vi "Diff_Drive_System_Dash_Write.vi"   [LabVIEW 2019]
uses:
  Diff_Drive_System_Globals.vi
  <vilib>/Rock Robotics/Network Tables/NT Write Numeric Array.vi
  <vilib>/Rock Robotics/Network Tables/NT Write Number.vi
  <vilib>/Rock Robotics/Network Tables/NT Write Boolean.vi
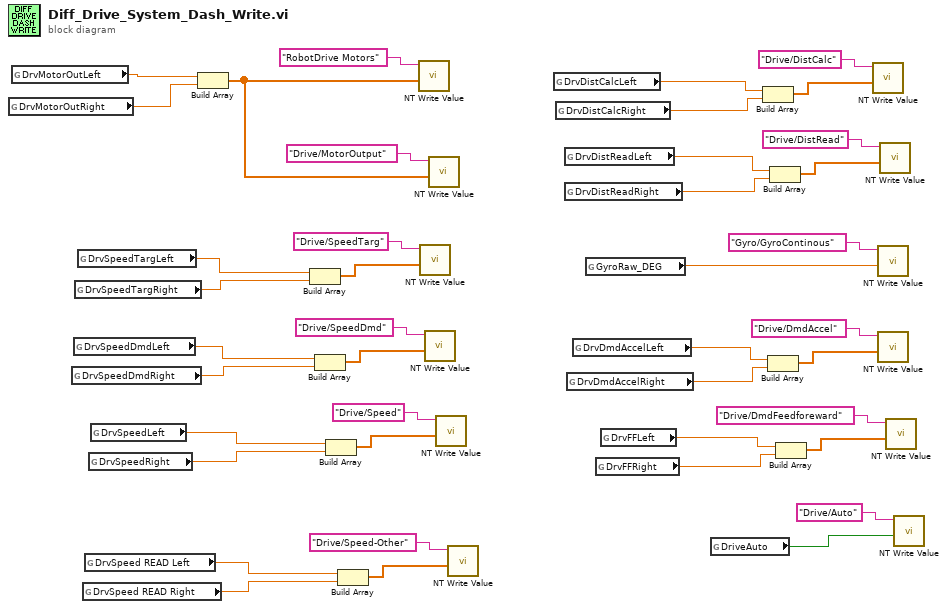
[diagram p0: block diagram]
diagram:
  n1 = global read "Diff_Drive_System_Globals.vi" "DrvMotorOutRight"() -> (w23:dbl)
  n2 = global read "Diff_Drive_System_Globals.vi" "DrvMotorOutLeft"() -> (w24:dbl)
  n3 = global read "Diff_Drive_System_Globals.vi" "DrvSpeedDmdRight"() -> (w18:dbl)
  n4 = global read "Diff_Drive_System_Globals.vi" "DrvSpeedDmdLeft"() -> (w19:dbl)
  n5 = global read "Diff_Drive_System_Globals.vi" "DrvSpeedTargRight"() -> (w20:dbl)
  n6 = global read "Diff_Drive_System_Globals.vi" "DrvSpeedTargLeft"() -> (w21:dbl)
  n7 = global read "Diff_Drive_System_Globals.vi" "DrvSpeed READ Right"() -> (w3:dbl)
  n8 = global read "Diff_Drive_System_Globals.vi" "DrvSpeed READ Left"() -> (w4:dbl)
  n9 = global read "Diff_Drive_System_Globals.vi" "DrvSpeedRight"() -> (w16:dbl)
  n10 = global read "Diff_Drive_System_Globals.vi" "DrvSpeedLeft"() -> (w17:dbl)
  n11 = Build Array(w24, w23) -> (w22:dbl[])
  n12 = Build Array(w21, w20) -> (w27:dbl[])
  n13 = Build Array(w19, w18) -> (w29:dbl[])
  n14 = Build Array(w17, w16) -> (w31:dbl[])
  n15 = Build Array(w4, w3) -> (w5:dbl[])
  n16 = call-poly <vilib>:"NT Write Value.vi"("Numeric Array"=w22, "Name"="RobotDrive Motors") -> ()  [unwired: 9 in, 1 out]
  n17 = call-poly <vilib>:"NT Write Value.vi"("Numeric Array"=w27, "Name"="Drive/SpeedTarg") -> ()  [unwired: 9 in, 1 out]
  n18 = call-poly <vilib>:"NT Write Value.vi"("Numeric Array"=w29, "Name"="Drive/SpeedDmd") -> ()  [unwired: 9 in, 1 out]
  n19 = call-poly <vilib>:"NT Write Value.vi"("Numeric Array"=w22, "Name"="Drive/MotorOutput") -> ()  [unwired: 9 in, 1 out]
  n20 = call-poly <vilib>:"NT Write Value.vi"("Numeric Array"=w31, "Name"="Drive/Speed") -> ()  [unwired: 9 in, 1 out]
  n21 = call-poly <vilib>:"NT Write Value.vi"("Numeric Array"=w5, "Name"="Drive/Speed-Other") -> ()  [unwired: 9 in, 1 out]
  n22 = global read "Diff_Drive_System_Globals.vi" "DrvDistCalcLeft"() -> (w15:dbl)
  n23 = global read "Diff_Drive_System_Globals.vi" "DrvDistCalcRight"() -> (w14:dbl)
  n24 = global read "Diff_Drive_System_Globals.vi" "DrvDistReadLeft"() -> (w13:dbl)
  n25 = global read "Diff_Drive_System_Globals.vi" "DrvDistReadRight"() -> (w12:dbl)
  n26 = global read "Diff_Drive_System_Globals.vi" "DrvDmdAccelRight"() -> (w9:dbl)
  n27 = global read "Diff_Drive_System_Globals.vi" "DrvDmdAccelLeft"() -> (w10:dbl)
  n28 = global read "Diff_Drive_System_Globals.vi" "GyroRaw_DEG"() -> (w11:dbl)
  n29 = global read "Diff_Drive_System_Globals.vi" "DrvFFRight"() -> (w7:dbl)
  n30 = global read "Diff_Drive_System_Globals.vi" "DrvFFLeft"() -> (w8:dbl)
  n31 = global read "Diff_Drive_System_Globals.vi" "DriveAuto"() -> (w1:bool)
  n32 = Build Array(w15, w14) -> (w33:dbl[])
  n33 = Build Array(w10, w9) -> (w38:dbl[])
  n34 = Build Array(w13, w12) -> (w35:dbl[])
  n35 = Build Array(w8, w7) -> (w40:dbl[])
  n36 = call-poly <vilib>:"NT Write Value.vi"("Numeric Array"=w33, "Name"="Drive/DistCalc") -> ()  [unwired: 9 in, 1 out]
  n37 = call-poly <vilib>:"NT Write Value.vi"("Numeric"=w11, "Name"="Gyro/GyroContinous") -> ()  [unwired: 9 in, 1 out]
  n38 = call-poly <vilib>:"NT Write Value.vi"("Numeric Array"=w38, "Name"="Drive/DmdAccel") -> ()  [unwired: 9 in, 1 out]
  n39 = call-poly <vilib>:"NT Write Value.vi"("Numeric Array"=w35, "Name"="Drive/DistRead") -> ()  [unwired: 9 in, 1 out]
  n40 = call-poly <vilib>:"NT Write Value.vi"("Numeric Array"=w40, "Name"="Drive/DmdFeedforeward") -> ()  [unwired: 9 in, 1 out]
  n41 = call-poly <vilib>:"NT Write Value.vi"("Boolean"=w1, "Name"="Drive/Auto") -> ()  [unwired: 9 in, 1 out]
